vi "Display.vi"(6 "test fail message":string="Test failed. Failure time: %s", 7 "test pass message":string="Test passed", 8 "error in":errorcluster, 11 "test results in":refnum<class "Test Results.lvclass">) -> (0 "error out":errorcluster)   [LabVIEW 2020, in "Test Results.lvclass"]
doc: "This VI displays a dialog that indicates the test results."
uses:
  Test Results.lvclass
  Test Results.lvclass/Test Results.ctl
panel:
  # "This Test Results class member VI displays a dialog that indicates the test results.\n\nYou can enter the message that will be displayed based on the result in the text controls \"test pass message\" and \"test fail message\"."
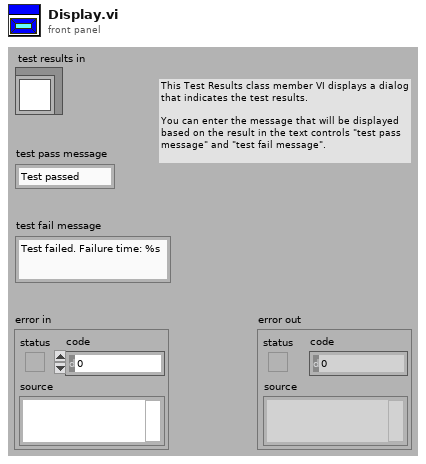
[diagram p1: front panel]
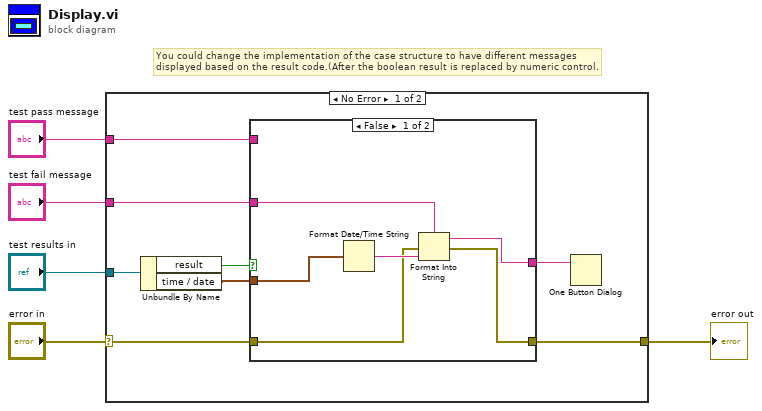
[diagram p0: block diagram]
diagram:
  # "You could change the implementation of the case structure to have different messages displayed based on the result code.(After the boolean result is replaced by numeric control."
  n1 = case shown="No Error" "error in" {
    selector: "error in" -> [w12 w22]
    tunnel: "test results in" -> [w11 _]
    tunnel: [w8 w22] -> w3
    tunnel: "test fail message" -> [w7 _]
    tunnel: "test pass message" -> [w6 _]
    frame No Error {
      n2 = Unbundle By Name(w11) -> ("result"=w13:bool, "time / date"=w10:timestamp)
      n3 = case shown="False" w13 {
        tunnel: w12 -> [w16 w21]
        tunnel: w10 -> [w19 _]
        tunnel: [w17 w20] -> w9
        tunnel: [w15 w21] -> w8
        tunnel: w7 -> [w14 _]
        tunnel: w6 -> [_ w20]
        frame False {
          n4 = Format Date/Time String(seconds (now)=w19) -> (date/time string=w18:string)  [unwired: 2 in]
          n5 = Format Into String(format string=w14, error in=w16, w18) -> (resulting string=w17:string, error out=w15:errorcluster)  [unwired: 1 in]
        }
        frame True {
        }
      }
      n6 = One Button Dialog(message=w9) -> ()  [unwired: 1 in, 1 out]
    }
    frame Error {
    }
  }
  "error out" <- w3
